vi "Parameter XML Write (Ballard-1533).vi"(6 "hw configuration":T1[](array[typedef]), 8 "error in":errorcluster caption="error out", 10 "Array":T2[](array[typedef]), 11 "parameter file in":refnum<k24>) -> (0 "error out":errorcluster, 3 "parameter file out":refnum<k24>)   [LabVIEW 2020]
uses:
  Libraries/Aim_1553_Parameter_ni/AIM_1553_Parameter_ni.lvlib
  Libraries/Aim_1553_Parameter_ni/_tyedefs/message_type.ctl
  Libraries/Aim_1553_Parameter_ni/_tyedefs/messageAddress_type.ctl
  _controls/1553_Parameters_key.ctl
  Libraries/Aim_1553_Parameter_ni/_tyedefs/parameter_type.ctl
  _controls/aim1553_messages.ctl
  _controls/1553_Parameters.ctl
  _controls/1553_minorFrames.ctl
  _controls/aim1553_cluster.ctl
  _controls/aim1553_RT_list.ctl
  C:/Users/Administrator/Desktop/GIT/Ballard-Arinc-429-XML-Generator/Source/Assemblies/Ballard_1553_Parameter_ni/bin/Debug/Ballard_1553_Parameter_ni.dll
  Assemblies/Ballard_1553_Parameter_ni/bin/Debug/Ballard_1553_Parameter_ni.dll
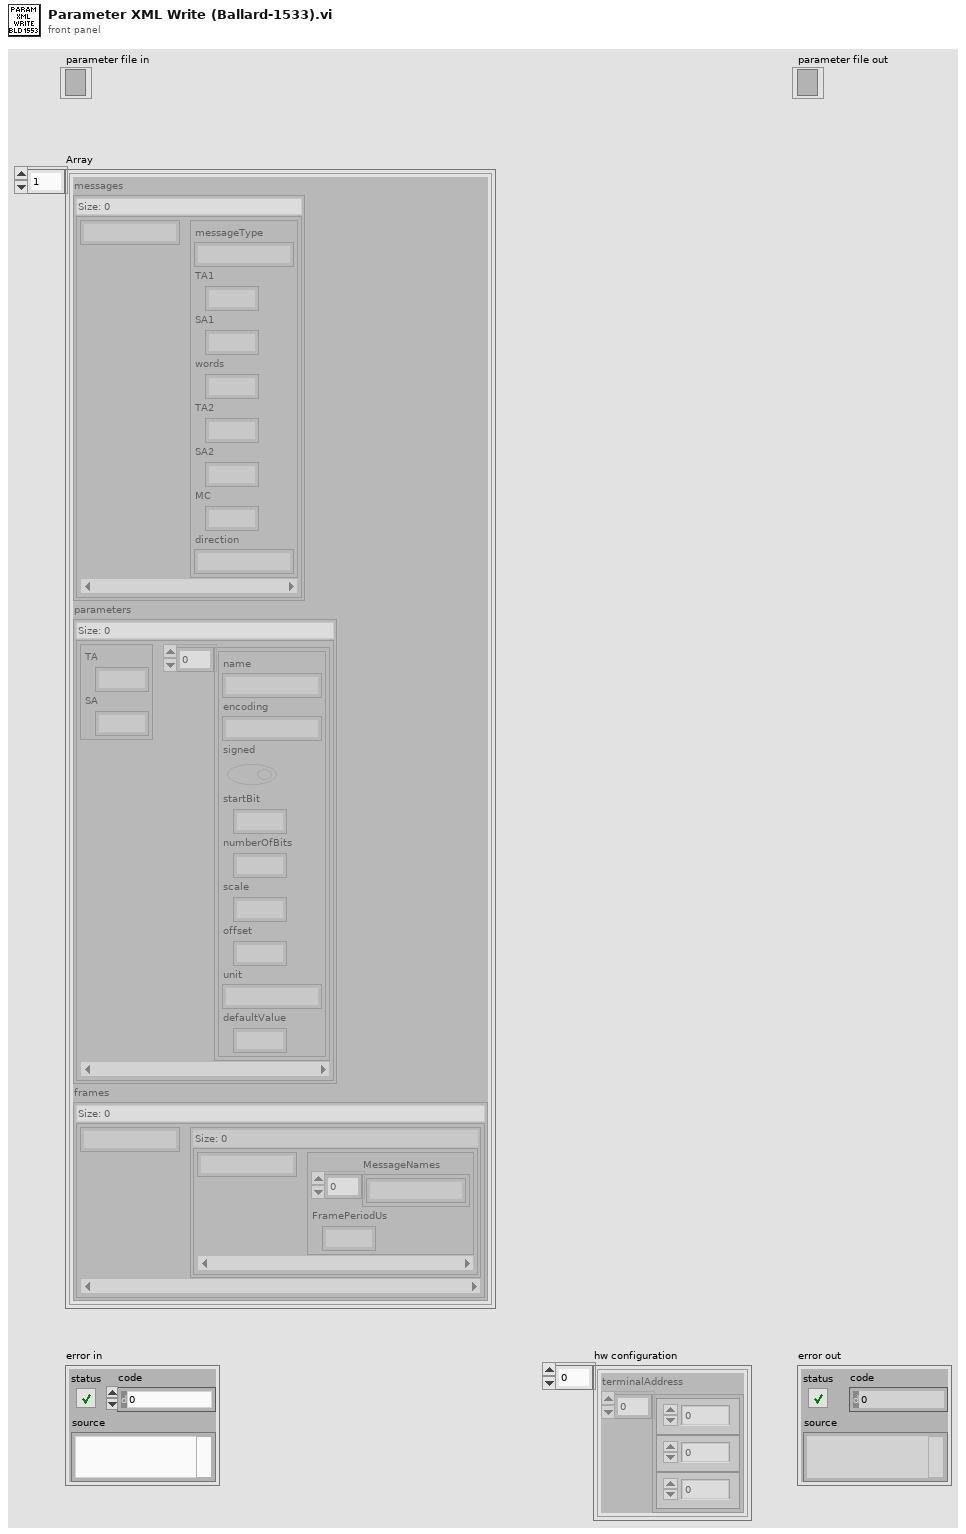
[diagram p1: front panel]
types:
  T1 = typedef "aim1553_RT_list.ctl" = cluster{"terminalAddress":i32[]}
  T2 = typedef "aim1553_cluster.ctl" = cluster{"messages":map{string, T3}, "parameters":map{T4, T5[]}, "frames":map{string, map{string, T6}}}
  T3 = typedef "aim1553_messages.ctl" = cluster{"messageType":string, "TA1":i32, "SA1":i32, "words":i32, "TA2":i32, "SA2":i32, "MC":i32, "direction":string}
  T4 = typedef "1553_Parameters_key.ctl" = cluster{"TA":i32, "SA":i32}
  T5 = typedef "1553_Parameters.ctl" = cluster{"name":string, "encoding":string, "signed":bool, "startBit":i32, "numberOfBits":i32, "scale":dbl, "offset":dbl, "unit":string, "defaultValue":dbl}
  T6 = typedef "1553_minorFrames.ctl" = cluster{"MessageNames":string[], "FramePeriodUs":i32}
  T7 = typedef "AIM_1553_Parameter_ni.lvlib/message_type.ctl" = cluster{"name":string, "numberOfWords":i32, "modeCode":i32, "messageType":i32, "createTimestampChannel":bool, "modeCodeSpecified":bool}
  T8 = typedef "AIM_1553_Parameter_ni.lvlib/parameter_type.ctl" = cluster{"defaultValue":dbl, "encoding":i32, "name":string, "numberOfBits":i32, "offset":dbl, "scale":dbl, "signed":bool, "startBit":i32, "unit":string}
  T9 = typedef "AIM_1553_Parameter_ni.lvlib/messageAddress_type.ctl" = cluster{"direction":i32, "subAddress":i32, "terminalAddress":i32}
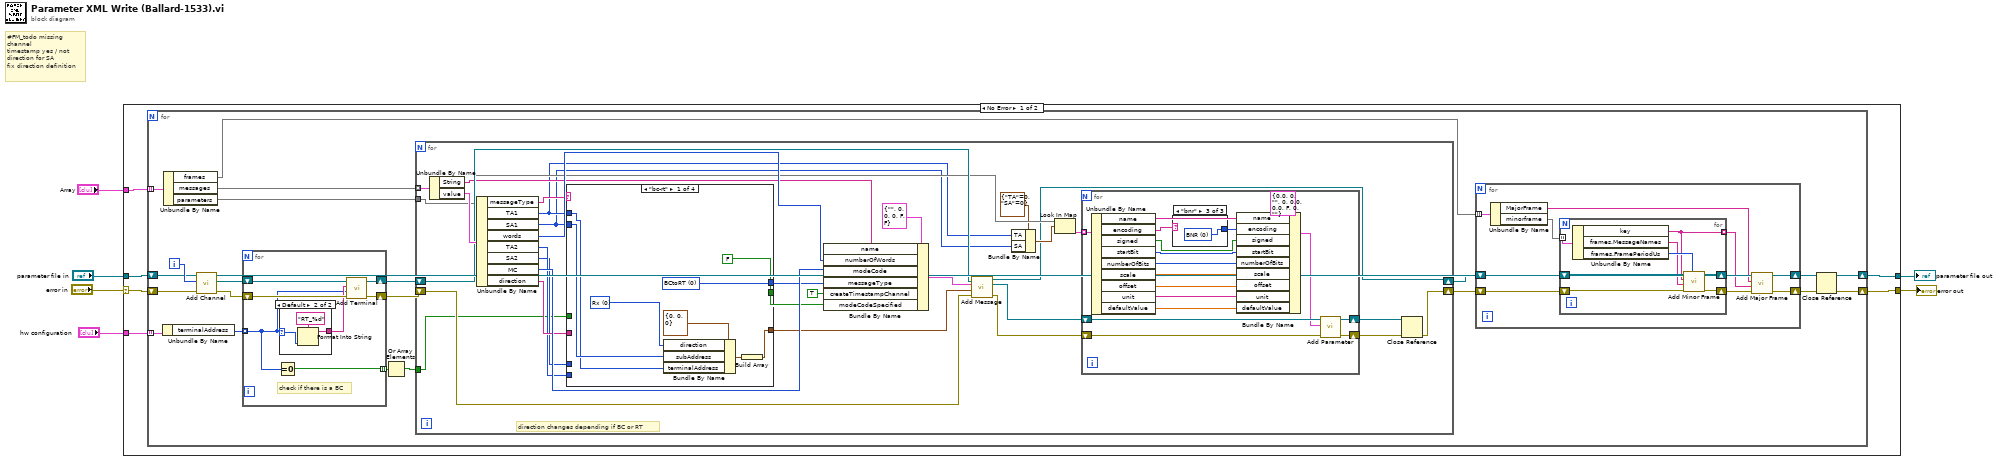
[diagram p0: block diagram]
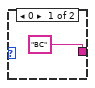
[diagram p2: hidden frame]
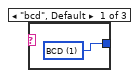
[diagram p3: hidden frame]
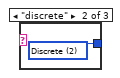
[diagram p4: hidden frame]
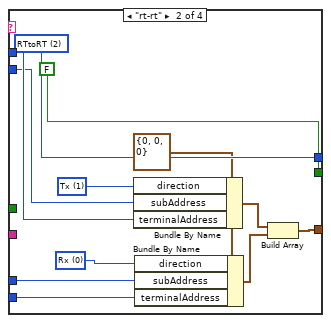
[diagram p5: hidden frame]
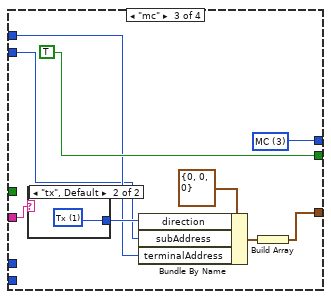
[diagram p6: hidden frame]
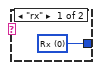
[diagram p7: hidden frame]
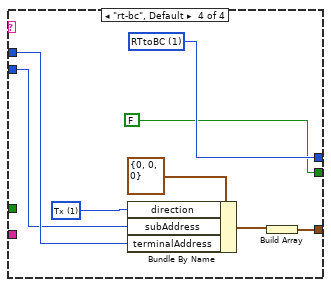
[diagram p8: hidden frame]
diagram:
  # "#FM_todo missing \nchannel\ntimestamp yes / not\ndirection for SA\nfix direction definition"
  n1 = case shown="No Error" "error in" {
    selector: "error in" -> [w11 w153]
    tunnel: "Array" -> [w10 _]
    tunnel: "parameter file in" -> [w12 w152]
    tunnel: [w8 w153] -> w3
    tunnel: [w9 w152] -> w2
    tunnel: "hw configuration" -> [w7 _]
    frame No Error {
      n2 = for {
        tunnel: w10 -> [w31] mode=indexing
        tunnel: w7 -> [w18] mode=indexing
        shift-right: [w29] -> w9
        shift-left: w12 -> [w13]
        shift-right: [w24] -> w8
        shift-left: w11 -> [w33]
        i -> [w16]
        n3 = Unbundle By Name(w18) -> ("terminalAddress"=w17:i32[])
        n4 = Unbundle By Name(w31) -> ("frames"=w19:map{string, map{string, T6}}, "messages"=w32:map{string, T3}, "parameters"=w30:map{T4, T5[]})
        n5 = call "Add Channel.vi"("error in"=w33, "hardwareChannel"=w16, "parameter file in"=w13) -> ("error out"=w28:errorcluster, "new channel"=w27:refnum<k24>, "parameter file out"=w29:refnum<k24>)  [unwired: 6 in]
        n6 = for {
          shift-right: [w38] -> w26
          shift-left: w28 -> [w40]
          shift-right: [w37] -> w25
          shift-left: w27 -> [w39]
          tunnel: w17 -> [w35] mode=indexing
          tunnel: [w34] -> w15 mode=indexing
          # "check if there is a BC"
          n7 = Equal To 0?(x=w35) -> (x = 0?=w34:bool)
          n8 = case shown="Default" w35 {
            selector: w35 -> [_ w43]
            tunnel: ["BC" ("BC") w44] -> w36
            frame 0 {
            }
            frame Default {
              n9 = Format Into String(format string="RT_%d", w43) -> (resulting string=w44:string)  [unwired: 2 in, 1 out]
            }
          }
          n10 = call "Add Terminal.vi"("error in"=w40, "terminalAddress"=w35, "name"=w36, "channel in"=w39) -> ("error out"=w38:errorcluster, "channel out"=w37:refnum<k24>)  [unwired: 5 in, 1 out]
        }
        n11 = Or Array Elements(Boolean array=w15) -> (logical OR=w14:bool)
        n12 = for {
          tunnel: w32 -> [w92] mode=indexing
          tunnel: w30 -> [w72]
          shift-right: [w64] -> w23
          shift-left: w25 -> [w89]
          shift-right: [w65] -> w22
          shift-left: w26 -> [w79]
          tunnel: w14 -> [w63]
          # "direction changes depending if BC or RT"
          n13 = Unbundle By Name(w92) -> ("String"=w71:string, "value"=w91:T3)
          n14 = Unbundle By Name(w91) -> ("messageType"=w86:string, "TA1"=w68:i32, "SA1"=w67:i32, "words"=w87:i32, "TA2"=w74:i32, "SA2"=w73:i32, "MC"=w85:i32, "direction"=w81:string)
          n15 = case shown="\"bc-rt\"" w86 {
            tunnel: [w120 w132 w141 w151] -> w83
            tunnel: [FALSE FALSE TRUE FALSE] -> w82
            tunnel: w81 -> [_ _ w137 _]
            tunnel: w68 -> [w116 w124 w135 w147]
            tunnel: w67 -> [w117 w123 w134 w146]
            tunnel: [w114 w126 w133 w144] -> w80
            tunnel: w74 -> [_ w122 _ _]
            tunnel: w73 -> [_ w121 _ _]
            tunnel: w63 -> [_ _ _ _]
            frame "bc-rt" {
              w113 = 0 items=["Rx", "Tx"] ("direction")
              w120 = 0 items=["BCtoRT", "RTtoBC", "RTtoRT", "MC"] ("messageType")
              n16 = Bundle By Name(cluster=T9 {"direction"=0, "subAddress"=0, "terminalAddress"=0} ("messageAddress"), "direction"=w113, "subAddress"=w117, "terminalAddress"=w116) -> (w115:T9)
              n17 = Build Array(w115) -> (w114:T9[])
            }
            frame "rt-rt" {
              w125 = 0 items=["Rx", "Tx"] ("direction")
              w130 = 1 items=["Rx", "Tx"] ("direction")
              w127 = T9 {"direction"=0, "subAddress"=0, "terminalAddress"=0} ("messageAddress")
              w132 = 2 items=["BCtoRT", "RTtoBC", "RTtoRT", "MC"] ("messageType")
              n18 = Bundle By Name(cluster=w127, "direction"=w130, "subAddress"=w123, "terminalAddress"=w124) -> (w129:T9)
              n19 = Bundle By Name(cluster=w127, "direction"=w125, "subAddress"=w121, "terminalAddress"=w122) -> (w128:T9)
              n20 = Build Array(w129, w128) -> (w126:T9[])
            }
            frame "mc" {
              w141 = 3 items=["BCtoRT", "RTtoBC", "RTtoRT", "MC"] ("messageType")
              n21 = case shown="\"tx\", Default" w137 {
                tunnel: [w142 w143] -> w136
                frame "rx" {
                  w142 = 0 items=["Rx", "Tx"] ("direction")
                }
                frame "tx", Default {
                  w143 = 1 items=["Rx", "Tx"] ("direction")
                }
              }
              n22 = Bundle By Name(cluster=T9 {"direction"=0, "subAddress"=0, "terminalAddress"=0} ("messageAddress"), "direction"=w136, "subAddress"=w134, "terminalAddress"=w135) -> (w138:T9)
              n23 = Build Array(w138) -> (w133:T9[])
            }
            frame "rt-bc", Default {
              w148 = 1 items=["Rx", "Tx"] ("direction")
              w151 = 1 items=["BCtoRT", "RTtoBC", "RTtoRT", "MC"] ("messageType")
              n24 = Bundle By Name(cluster=T9 {"direction"=0, "subAddress"=0, "terminalAddress"=0} ("messageAddress"), "direction"=w148, "subAddress"=w146, "terminalAddress"=w147) -> (w145:T9)
              n25 = Build Array(w145) -> (w144:T9[])
            }
          }
          n26 = Bundle By Name(cluster=T7 {"name"="", "numberOfWords"=0, "modeCode"=0, "messageType"=0, "createTimestampChannel"=FALSE, "modeCodeSpecified"=FALSE} ("message configuration"), "name"=w71, "numberOfWords"=w87, "modeCode"=w85, "messageType"=w83, "createTimestampChannel"=TRUE, "modeCodeSpecified"=w82) -> (w88:T7)
          n27 = call "Add Message.vi"("error in"=w79, "messageAddresses"=w80, "message configuration"=w88, "channel in"=w89) -> ("error out"=w78:errorcluster, "new message"=w77:refnum<k24>, "channel out"=w64:refnum<k24>)  [unwired: 5 in]
          n28 = Bundle By Name(cluster=T4 {"TA"=0, "SA"=0} ("key"), "TA"=w68, "SA"=w67) -> (w69:T4)
          n29 = Look In Map(map=w72, key=w69) -> (value=w66:T5[])  [unwired: 1 in, 1 out]
          n30 = for {
            shift-right: [w106] -> w75
            shift-left: w78 -> [w109]
            shift-right: [w107] -> w76
            shift-left: w77 -> [w108]
            tunnel: w66 -> [w104] mode=indexing
            n31 = Unbundle By Name(w104) -> ("name"=w102:string, "encoding"=w101:string, "signed"=w99:bool, "startBit"=w98:i32, "numberOfBits"=w97:i32, "scale"=w96:dbl, "offset"=w95:dbl, "unit"=w94:string, "defaultValue"=w93:dbl)
            n32 = case shown="\"bnr\"" w101 {
              tunnel: [w110 w111 w112] -> w100
              frame "bcd", Default {
                w110 = 1 items=["BNR", "BCD", "Discrete"] ("encoding")
              }
              frame "discrete" {
                w111 = 2 items=["BNR", "BCD", "Discrete"] ("encoding")
              }
              frame "bnr" {
                w112 = 0 items=["BNR", "BCD", "Discrete"] ("encoding")
              }
            }
            n33 = Bundle By Name(cluster=T8 {"defaultValue"=0.0, "encoding"=0, "name"="", "numberOfBits"=0, "offset"=0.0, "scale"=0.0, "signed"=FALSE, "startBit"=0, "unit"=""} ("parameter configuration"), "name"=w102, "encoding"=w100, "signed"=w99, "startBit"=w98, "numberOfBits"=w97, "scale"=w96, "offset"=w95, "unit"=w94, "defaultValue"=w93) -> (w103:T8)
            n34 = call "Add Parameter.vi"("error in"=w109, "parameter configuration"=w103, "message in"=w108) -> ("error out"=w106:errorcluster, "message out"=w107:refnum<k24>)  [unwired: 6 in, 1 out]
          }
          n35 = Close Reference(reference=w76, error in (no error)=w75) -> (error out=w65:errorcluster)
        }
        n36 = for {
          shift-right: [w54] -> w21
          shift-left: w23 -> [w50]
          shift-right: [w53] -> w20
          shift-left: w22 -> [w48]
          tunnel: w19 -> [w52] mode=indexing
          n37 = Unbundle By Name(w52) -> ("MajorFrame"=w51:string, "minorframe"=w46:map{string, T6})
          n38 = for {
            shift-right: [w61] -> w49
            shift-left: w50 -> [w58]
            shift-right: [w60] -> w47
            shift-left: w48 -> [w57]
            tunnel: w46 -> [w62] mode=indexing
            tunnel: [w55] -> w45 mode=indexing
            n39 = Unbundle By Name(w62) -> ("key"=w55:string, "frames.MessageNames"=w56:string[], "frames.FramePeriodUs"=w59:i32)
            n40 = call "Add Minor Frame.vi"("minorFramePeriod"=w59, "error in"=w57, "messageRefs"=w56, "name"=w55, "channel in"=w58) -> ("error out"=w60:errorcluster, "channel out"=w61:refnum<k24>)  [unwired: 4 in, 1 out]
          }
          n41 = call "Add Major Frame.vi"("error in"=w47, "minorFrameNames"=w45, "name"=w51, "channel in"=w49) -> ("error out"=w53:errorcluster, "channel out"=w54:refnum<k24>)  [unwired: 5 in, 1 out]
        }
        n42 = Close Reference(reference=w21, error in (no error)=w20) -> (error out=w24:errorcluster)
      }
    }
    frame Error {
    }
  }
  "error out" <- w3
  "parameter file out" <- w2
